vi "Launcher.vi"   [LabVIEW 2020]
uses:
  Real Hardware/Microscope_RM21/Microscope_RM21/Microscope_RM21.lvclass
  C:/Program Files/National Instruments/LabVIEW 2020/vi.lib/ActorFramework/Actor/Actor.lvclass
  <vilib>/ActorFramework/Actor/Actor.lvclass
panel:
  # "MMicroscope"
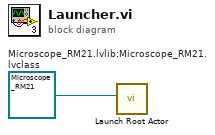
[diagram p0: block diagram]
diagram:
  w1 = refnum<class "Microscope_RM21.lvclass"> refnum  # Microscope_RM21.lvlib:Microscope_RM21.lvclass
  n1 = call <vilib>:"Launch Root Actor.vi"("Actor"=w1) -> ()  [unwired: 9 in, 2 out]
